vi "LV FPGA Serial Read.vi"(1 "Read FIFO":refnum<k21>="Read FIFO", 5 "Receive":refnum<k21>="Port8/DIOCTL", 7 "baud rate (9600)":u32=9600, 9 "data bits (8)":i32=8 min=5 max=8 step=1, 11 "parity (0:none)":enum16{"None", "Odd", "Even", "Mark", "Space"}(ring), 12 "stop bits (10: 1 bit)":u16(ring)=10 items=["1.0"=10, "1.5"=15, "2.0"=20], 13 "Invert Polarity?":bool) -> ()   [LabVIEW 2009]
uses:
  <vilib>/eio/EIONode/EIONode.xnode
  <vilib>/rvi/eio/nirviEIOImplementation/nirviEIOImplementation.xnode
  <vilib>/rvi/eio/common/nirviEmuTemplateMethod_noerrors.vi
  <vilib>/rvi/eio/common/nirviEmuClasses.ctl
  Instance           1 27Saved   LV FPGA Serial Read .vi
  Instance           2 27Saved   LV FPGA Serial Read .vi
  <vilib>/rvi/DataTransferAndStorage/Container/XNode/niFpgaContainer.xnode
  <vilib>/rvi/DataTransferAndStorage/Container/Common/niFpgaContainerMethod.ctl
  <vilib>/rvi/DataTransferAndStorage/Container/Common/niFpgaContainerExecOnDevCompGetState.vi
  <vilib>/rvi/DataTransferAndStorage/Container/Common/niFpgaContainerMetaDataKey.ctl
  <vilib>/rvi/FIFO/Fifo_Resource/nirvififoUniquifyingName.vi
  <vilib>/rvi/interface/RandomDataEmulation/niFpgaRandomDataHandleErrors.vi
  <vilib>/rvi/interface/RandomDataEmulation/nirviRandomDataFPGAFIFO.vi
  <vilib>/rvi/DataTransferAndStorage/Container/Common/niFpgaTransferTypeControl.ctl
  <vilib>/rvi/DataTransferAndStorage/FIFO/niFpgaPeerToPeerStreamState.ctl
  <vilib>/rvi/eio/common/nirviEmuReportErrorAndStop.vi
  Instance           3 27Saved   LV FPGA Serial Read .vi
  Instance           6 27Saved   LV FPGA Serial Read .vi
panel:
  out "Read: Transmission Error":bool
  in  "stop":bool
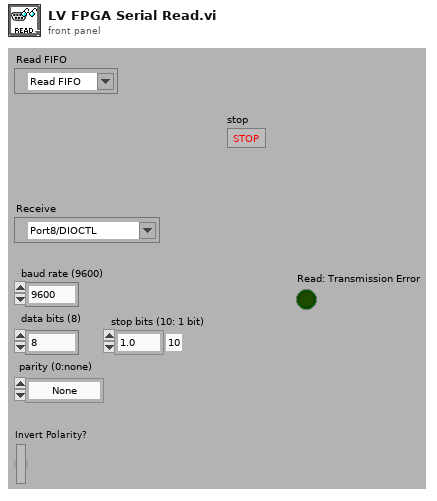
[diagram p1: front panel]
types:
  T1 = typedef "nirviEmuClasses.ctl" = enum16{"IO Read", "IO Write", "Method", "Property Read", "Property Write"}
  T2 = typedef "niFpgaContainerMethod.ctl" = enum16{"Write", "Read", "Clear", "Get Number of Elements to Write", "Get Number of Elements to Read", "Enable", "Disable", "Flush and Disable", "Get Stream State"}
  T3 = typedef "niFpgaTransferTypeControl.ctl" = enum16{"Target-Scoped", "Host to Target - DMA", "Target to Host - DMA", "Peer to Peer Reader", "Peer to Peer Writer", "Bidirectional"}
  T4 = typedef "niFpgaPeerToPeerStreamState.ctl" = enum16{"Unlinked", "Disabled", "Enabled", "Flushing"}
  T5 = typedef "niFpgaContainerMetaDataKey.ctl" = enum16{"FPGA FIFO", "FPGA Memory", "FPGA Register"}
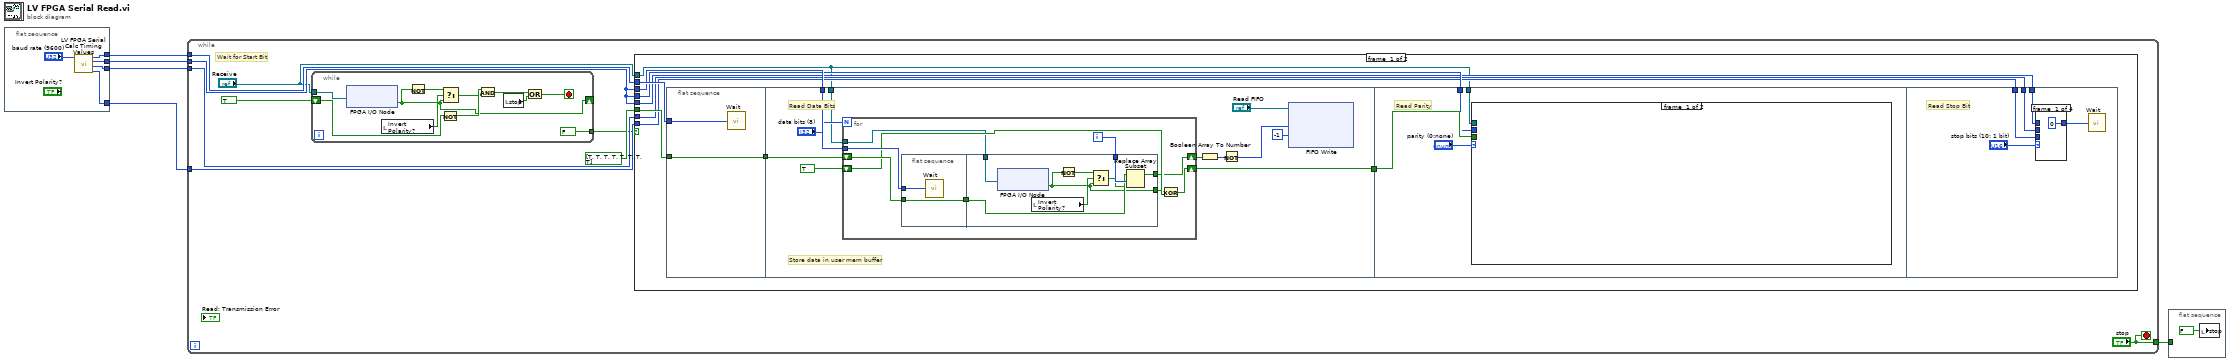
[diagram p0: block diagram]
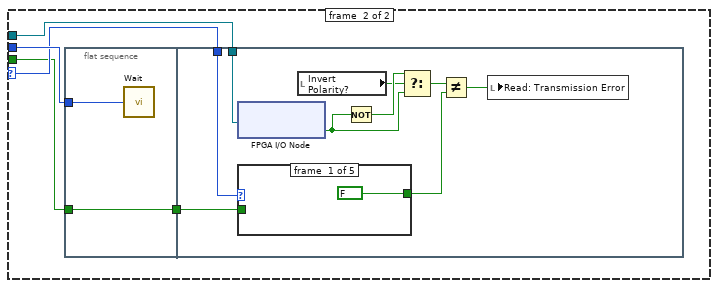
[diagram p2: hidden frame]
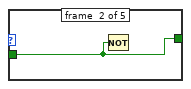
[diagram p3: hidden frame]
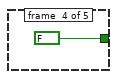
[diagram p5: hidden frame]
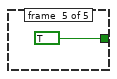
[diagram p6: hidden frame]
diagram:
  n1 = flat-sequence {
    tunnel: [w6] -> w4
    tunnel: [w9] -> w5
    tunnel: [w8] -> w3
    tunnel: [w7] -> w2
    frame #0 {
      n2 = call "LV FPGA Serial Calc Timing Values.vi"("baud rate (1000000)"="baud rate (9600)") -> ("Two Bit"=w7:u32, "One and Half Bit"=w8:u32, "One Bit"=w6:u32, "Half Bit"=w9:u32)  [unwired: 1 in, 2 out]
    }
  }
  n3 = while {
    tunnel: w2 -> [w18]
    tunnel: w3 -> [w17]
    tunnel: w4 -> [w16]
    tunnel: w5 -> [w15]
    tunnel: ["stop"] -> w1
    stop <- "stop" stop-if-true
    # "Wait for Start Bit"
    n4 = while {
      tunnel: [FALSE] -> w14
      shift-right: [w20] -> _
      shift-left: TRUE -> [w29]
      tunnel: "Receive" -> [w24]
      stop <- w25 stop-if-true
      n5 = xnode "FPGA I/O Node"("FPGA I/O In"=w24) -> ("I/O Item"=w20:bool)  [unwired: 1 out]
      n6 = local read "Invert Polarity?"() -> (w22:bool)
      n7 = Not(x=w20) -> (.not. x?=w23:bool)
      n8 = Not(x=w29) -> (.not. x?=w28:bool)
      n9 = Select(t=w23, s=w22, f=w20) -> (s? t:f=w21:bool)
      n10 = And(x=w28, y=w21) -> (x .and. y?=w26:bool)
      n11 = local read "stop"() -> (w27:bool)
      n12 = Or(x=w26, y=w27) -> (x .or. y?=w25:bool)
    }
    n13 = case shown="False" w14 {
      tunnel: bool[] [TRUE, TRUE, TRUE, TRUE, TRUE, TRUE, TRUE, TRUE] -> [w60 _]
      tunnel: w15 -> [w59 _]
      tunnel: w16 -> [w58 _]
      tunnel: w16 -> [w57 _]
      tunnel: w16 -> [w56 _]
      tunnel: w17 -> [w55 _]
      tunnel: w18 -> [w54 _]
      tunnel: "Receive" -> [w52 _]
      frame #0 {
        n14 = flat-sequence {
          tunnel: [w63] -> w61
          tunnel: w60 -> [w63]
          tunnel: w59 -> [w62]
          tunnel: w61 -> [w74]
          tunnel: w58 -> [w73]
          tunnel: [w69] -> w53
          tunnel: w52 -> [w67]
          tunnel: w57 -> [w402]
          tunnel: w53 -> [w404]
          tunnel: w52 -> [w401]
          tunnel: w56 -> [w450]
          tunnel: w55 -> [w449]
          tunnel: w54 -> [w448]
          frame #0 {
            n15 = call "Wait"("Count(Ticks)"=w62) -> ()  [unwired: 1 out]
          }
          frame #1 {
            # "Store data in user mem buffer"
            # "Read Data Bits"
            n16 = for {
              N: "data bits (8)" -> [_]
              shift-right: [w363] -> w72
              shift-left: w74 -> [w369]
              tunnel: w73 -> [w367]
              shift-right: [w366] -> w69
              shift-left: TRUE -> [w365]
              tunnel: w67 -> [w361]
              i -> [w362]
              n17 = flat-sequence {
                tunnel: w369 -> [w371]
                tunnel: [w371] -> w368
                tunnel: w367 -> [w370]
                tunnel: w362 -> [w379]
                tunnel: w368 -> [w378]
                tunnel: [w377] -> w363
                tunnel: [w372] -> w364
                tunnel: w361 -> [w376]
                frame #0 {
                  n18 = call "Wait"("Count(Ticks)"=w370) -> ()  [unwired: 1 out]
                }
                frame #1 {
                  n19 = xnode "FPGA I/O Node"("FPGA I/O In"=w376) -> ("I/O Item"=w372:bool)  [unwired: 1 out]
                  n20 = local read "Invert Polarity?"() -> (w375:bool)
                  n21 = Not(x=w372) -> (.not. x?=w374:bool)
                  n22 = Select(t=w374, s=w375, f=w372) -> (s? t:f=w373:bool)
                  n23 = Replace Array Subset(array=w378, new element=w373, index=w379) -> (w377:bool[])
                }
              }
              n24 = Exclusive Or(1:w365, 2:w364) -> (0:w366:bool)
            }
            n25 = Boolean Array To Number(Boolean array=w72) -> (number=w71:u8)
            n26 = Not(x=w71) -> (.not. x?=w66:u8)
            n27 = xnode ("FIFO Write")("Element"=w66, "Timeout"=-1, "FIFO In"="Read FIFO") -> ()  [unwired: 2 out]
          }
          frame #2 {
            # "Read Parity"
            n28 = case shown="\"Odd\", Default" "parity (0:none)" {
              selector: "parity (0:none)" -> [_ w408]
              tunnel: w404 -> [_ w406]
              tunnel: w402 -> [_ w409]
              tunnel: w401 -> [_ w405]
              frame #0 {
              }
              frame #1 {
                n29 = flat-sequence {
                  tunnel: w409 -> [w411]
                  tunnel: [w410] -> w407
                  tunnel: w406 -> [w410]
                  tunnel: w408 -> [w420]
                  tunnel: w407 -> [w418]
                  tunnel: w405 -> [w416]
                  frame #0 {
                    n30 = call "Wait"("Count(Ticks)"=w411) -> ()  [unwired: 1 out]
                  }
                  frame #1 {
                    n31 = xnode "FPGA I/O Node"("FPGA I/O In"=w416) -> ("I/O Item"=w413:bool)  [unwired: 1 out]
                    n32 = case shown="\"None\"" w420 {
                      tunnel: w418 -> [_ w443 w444 _ _]
                      tunnel: [FALSE ("y") w443 w444 FALSE ("y") TRUE ("y")] -> w419
                      frame #0 {
                      }
                      frame #1 {
                        n33 = Not(x=w443) -> ()  [unwired: 1 out]
                      }
                      frame #2 {
                      }
                      frame #3 {
                      }
                      frame #4 {
                      }
                    }
                    n34 = local read "Invert Polarity?"() -> (w414:bool)
                    n35 = Not(x=w413) -> (.not. x?=w415:bool)
                    n36 = Select(t=w415, s=w414, f=w413) -> (s? t:f=w412:bool)
                    n37 = Not Equal?(x=w412, y=w419) -> (x != y?=w417:bool)
                    n38 = local write "Read: Transmission Error"(w417) -> ()
                  }
                }
              }
            }
          }
          frame #3 {
            # "Read Stop Bit"
            n39 = case shown="10" "stop bits (10: 1 bit)" {
              tunnel: w450 -> [_ w453 _ _]
              tunnel: w449 -> [_ _ w454 _]
              tunnel: w448 -> [_ _ _ w455]
              tunnel: [u32 0 ("One Bit") w453 w454 w455] -> w447
              frame #0 {
              }
              frame #1 {
              }
              frame #2 {
              }
              frame #3 {
              }
            }
            n40 = call "Wait"("Count(Ticks)"=w447) -> ()  [unwired: 1 out]
          }
        }
      }
      frame #1 {
      }
    }
  }
  n41 = flat-sequence {
    tunnel: w1 -> [_]
    frame #0 {
      n42 = local write "stop"(FALSE ("stop")) -> ()
    }
  }
